vi "RectangleComparisonGear.vi"(6 "Line Border":cluster{"Top":dbl, "Bottom":dbl}={"Top"=6.0, "Bottom"=1.0}, 9 "Second":dbl[](array[numeric]), 11 "First":dbl[](array[numeric])) -> (0 "Rect":T1, 1 "Line":T1, 3 "Scores":T2)   [LabVIEW 2016]
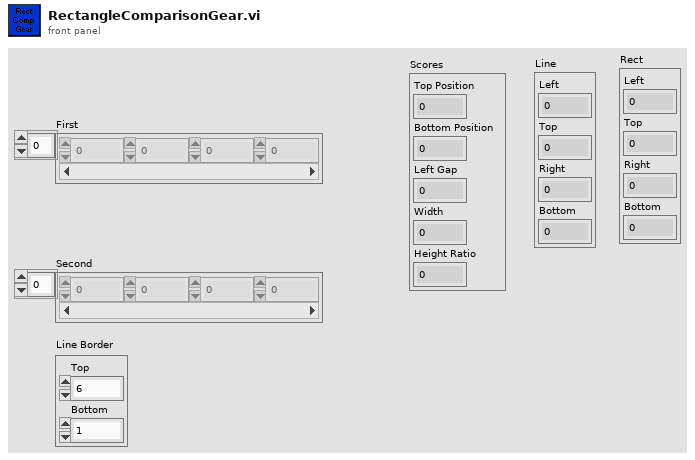
[diagram p1: front panel]
types:
  T1 = cluster{"Left":dbl, "Top":dbl, "Right":dbl, "Bottom":dbl}
  T2 = cluster{"Top Position":dbl, "Bottom Position":dbl, "Left Gap":dbl, "Width":dbl, "Height Ratio":dbl}
  T3 = cluster{"[0]":dbl, "[1]":dbl, "[2]":dbl, "[3]":dbl}
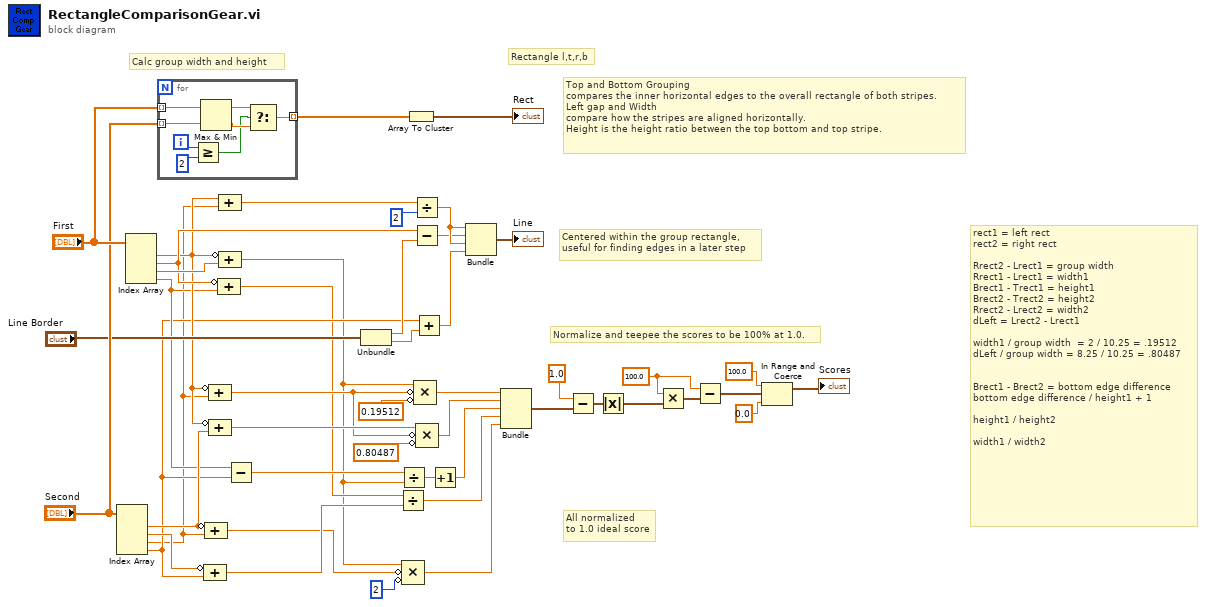
[diagram p0: block diagram]
diagram:
  w27 = 100.0 ("x/y")
  # "rect1 = left rect\nrect2 = right rect\n\nRrect2 - Lrect1 = group width\nRrect1 - Lrect1 = width1\nBrect1 - Trect1 = height1\nBrect2 - Trect2 = height2\nRrect2 - Lrect2 = width2\ndLeft = Lrect2 - Lrect1\n\nwidth1 / group width  = 2 / 10.25 = .19512\ndLeft / group width = 8.25 / 10.25 = .80487\n\n\nBrect1 - Brect2 = bottom edge difference\nbottom edge difference / height1 + 1\n\nheight1 / height2\n\nwidth1 / width2"
  # "Centered within the group rectangle,\nuseful for finding edges in a later step"
  # "All normalized\nto 1.0 ideal score"
  # "Normalize and teepee the scores to be 100% at 1.0."
  # "Top and Bottom Grouping\ncompares the inner horizontal edges to the overall rectangle of both stripes.\nLeft gap and Width\ncompare how the stripes are aligned horizontally.\nHeight is the height ratio between the top bottom and top stripe."
  # "Calc group width and height"
  # "Rectangle l,t,r,b"
  n1 = Index Array(array="Second") -> (element #1=w8:dbl, element #2=w19:dbl, element #3=w1:dbl, element #4=w6:dbl)  [unwired: 4 in]
  n2 = Index Array(array="First") -> (element #1=w9:dbl, element #2=w18:dbl, element #3=w42:dbl, element #4=w7:dbl)  [unwired: 4 in]
  n3 = for {
    tunnel: "First" -> [w55] mode=indexing
    tunnel: "Second" -> [w54] mode=indexing
    tunnel: [w48] -> w34 mode=indexing
    i -> [w52]
    n4 = Greater Or Equal?(x=w52, y=2) -> (x >= y?=w49:bool)
    n5 = Max & Min(x=w55, y=w54) -> (max(x,y)=w51:dbl, min(x,y)=w50:dbl)
    n6 = Select(t=w51, s=w49, f=w50) -> (s? t:f=w48:dbl)
  }
  n7 = Compound Arithmetic op=ADD(invert w19, w6) -> (w4:dbl)
  n8 = Compound Arithmetic op=ADD(invert w8, w1) -> (w2:dbl)
  n9 = Compound Arithmetic op=ADD(invert w9, w1) -> (w16:dbl)
  n10 = Compound Arithmetic op=ADD(invert w9, w8) -> (w17:dbl)
  n11 = Compound Arithmetic op=ADD(invert w18, w7) -> (w5:dbl)
  n12 = Compound Arithmetic op=ADD(w9, w1) -> (w41:dbl)
  n13 = Compound Arithmetic op=ADD(invert w9, w42) -> (w3:dbl)
  n14 = Subtract(x=w7, y=w6) -> (x-y=w47:dbl)
  n15 = Unbundle("Line Border") -> ("Top"=w10:dbl, "Bottom"=w11:dbl)
  n16 = Divide(x=w5, y=w4) -> (x/y=w45:dbl)
  n17 = Divide(x=w47, y=w3) -> (x/y=w43:dbl)
  n18 = Compound Arithmetic op=MULTIPLY(w3, invert w2, invert 2) -> (w44:dbl)
  n19 = Array To Cluster(array=w34) -> (cluster=→"Rect":T3)
  n20 = Divide(x=w41, y=2) -> (x/y=w40:dbl)
  n21 = Subtract(x=w18, y=w10) -> (x-y=w38:dbl)
  n22 = Add(x=w6, y=w11) -> (x+y=w32:dbl)
  n23 = Compound Arithmetic op=MULTIPLY(w3, invert w16, invert 0.19512 ("y")) -> (w46:dbl)
  n24 = Compound Arithmetic op=MULTIPLY(w17, invert w16, invert 0.80487 ("y")) -> (w15:dbl)
  n25 = Increment(x=w43) -> (x+1=w31:dbl)
  n26 = Bundle(w40, w38, w40, w32) -> (→"Line":cluster{dbl, dbl, dbl, dbl})  [unwired: 1 in]
  n27 = Bundle(w46, w15, w31, w45, w44) -> (w21:cluster{dbl, dbl, dbl, dbl, dbl})  [unwired: 1 in]
  n28 = Subtract(x=1.0 ("y"), y=w21) -> (x-y=w25:cluster{dbl, dbl, dbl, dbl, dbl})
  n29 = Absolute Value(x=w25) -> (abs(x)=w28:cluster{dbl, dbl, dbl, dbl, dbl})
  n30 = Multiply(x=w27, y=w28) -> (x*y=w29:cluster{dbl, dbl, dbl, dbl, dbl})
  n31 = Subtract(x=w27, y=w29) -> (x-y=w24:cluster{dbl, dbl, dbl, dbl, dbl})
  n32 = In Range and Coerce(upper limit=100.0, x=w24, lower limit=0.0) -> (coerced(x)=→"Scores":cluster{dbl, dbl, dbl, dbl, dbl})  [unwired: 1 out]
